vi "TDC_getLastTimestamps.vi"(8 "Error In":errorcluster, 10 "Buffer Size":i32, 11 "Reset":bool) -> (0 "Error Out":errorcluster, 1 "Channel Numbers":i8[](array[numeric]), 2 "Timestamps":i64[](array[numeric]), 3 "Valid Data":i32)   [LabVIEW 2011]
uses:
  dist/userlib/lib/tdcbase.dll
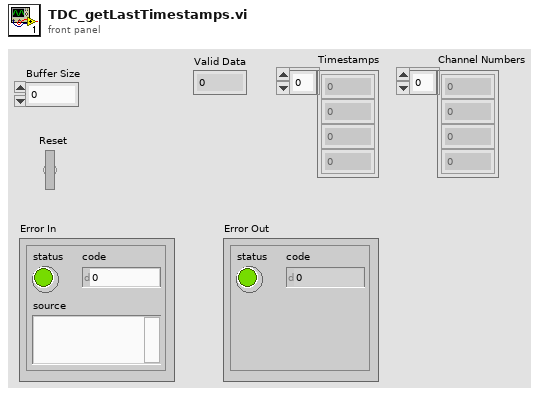
[diagram p1: front panel]
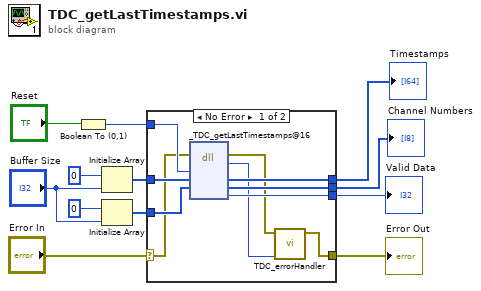
[diagram p0: block diagram]
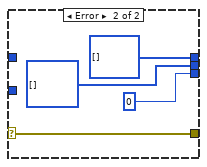
[diagram p2: hidden frame]
diagram:
  n1 = Boolean To (0,1)(Boolean="Reset") -> (0, 1=w6:i16)
  n2 = Initialize Array(i64 0, "Buffer Size") -> (w8:i64[])
  n3 = Initialize Array(i8 0, "Buffer Size") -> (w2:i8[])
  n4 = case shown="No Error" "Error In" {
    selector: "Error In" -> [w16 w26]
    tunnel: [w13 w26] -> w11
    tunnel: [w22 i64[] []] -> w10
    tunnel: w8 -> [w21 _]
    tunnel: w6 -> [w20 _]
    tunnel: [w19 0] -> w5
    tunnel: w2 -> [w18 _]
    tunnel: [w17 i8[] []] -> w1
    frame No Error {
      n5 = dll-call lib="C:/nh/projekt/spmctrl/dist/userlib/lib/tdcbase.dll" fn="_TDC_getLastTimestamps@16"(error in=w16, "reset"=w20, "timestamps"=w21, "channels"=w18) -> (error out=w15:errorcluster, "return type"=w14:i32, "timestamps"=w22:i64[], "channels"=w17:i8[], "valid"=w19:i32)  [unwired: 4 in, 1 out]
      n6 = call "TDC_errorHandler.vi"("quTAU Return Code"=w14, "Error In"=w15) -> ("Error Out"=w13:errorcluster)  [unwired: 9 in]
    }
    frame Error {
    }
  }
  "Error Out" <- w11
  "Timestamps" <- w10
  "Valid Data" <- w5
  "Channel Numbers" <- w1
